vi "setMenu.vi"(8 "flatMenu[]":T1, 11 "MenuRef":refnum<k9>) -> ()   [LabVIEW 2013]
uses:
  flatMenu.ctl
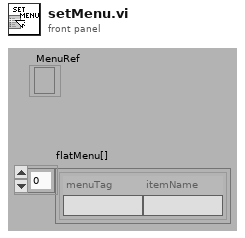
[diagram p1: front panel]
types:
  T1 = typedef "flatMenu.ctl" = cluster{"menuTag":string, "itemName":string}[]
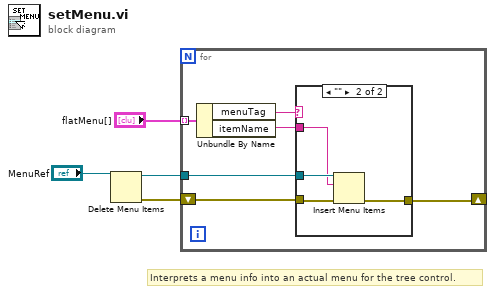
[diagram p0: block diagram]
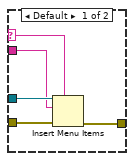
[diagram p2: hidden frame]
diagram:
  # "Interprets a menu info into an actual menu for the tree control."
  n1 = Delete Menu Items(9:"MenuRef") -> (0:w3:errorcluster, 3:w2:refnum<k9>)  [unwired: 3 in]
  n2 = for {
    tunnel: "flatMenu[]" -> [w10] mode=indexing
    tunnel: w2 -> [w7]
    shift-right: [w5] -> _
    shift-left: w3 -> [w6]
    n3 = Unbundle By Name(w10) -> ("menuTag"=w9:string, "itemName"=w8:string)
    n4 = case shown="\"\"" w9 {
      selector: w9 -> [w14 _]
      tunnel: w8 -> [w13 w18]
      tunnel: w7 -> [w15 w19]
      tunnel: w6 -> [w12 w16]
      tunnel: [w11 w17] -> w5
      frame Default {
        n5 = Insert Menu Items(5:w14, 6:w12, 8:w13, 9:w15) -> (0:w11:errorcluster)  [unwired: 2 in, 2 out]
      }
      frame "" {
        n6 = Insert Menu Items(6:w16, 8:w18, 9:w19) -> (0:w17:errorcluster)  [unwired: 3 in, 2 out]
      }
    }
  }
